vi "OP300ZP_SCANequipements.vi"(8 "Errin":errorcluster caption="errin", 10 "Chaîne":string="Log et conf\\Config.ini", 11 "pathin":path=path "D:/CODE/02 SLIM ZEN") -> (0 "ERROUT":errorcluster caption="error out", 1 "KO?":bool=TRUE, 3 "VISA OUT":T1)   [LabVIEW 2020]
doc: "Ce vi il détecte la presence des équipements"
uses:
  OP300-CONTI-AUTO/VG/VG_ATEQ.vi
  VG/VG_ST5520.vi
  VG/VG_BT3562.vi
  VG/VG_MX5060.vi
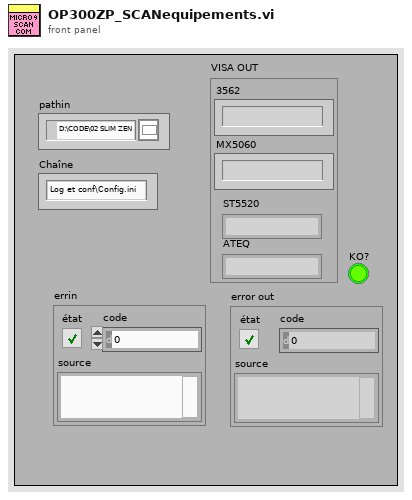
[diagram p1: front panel]
types:
  T1 = cluster{"3562":string, "MX5060":string, "ST5520":string, "ATEQ":string}
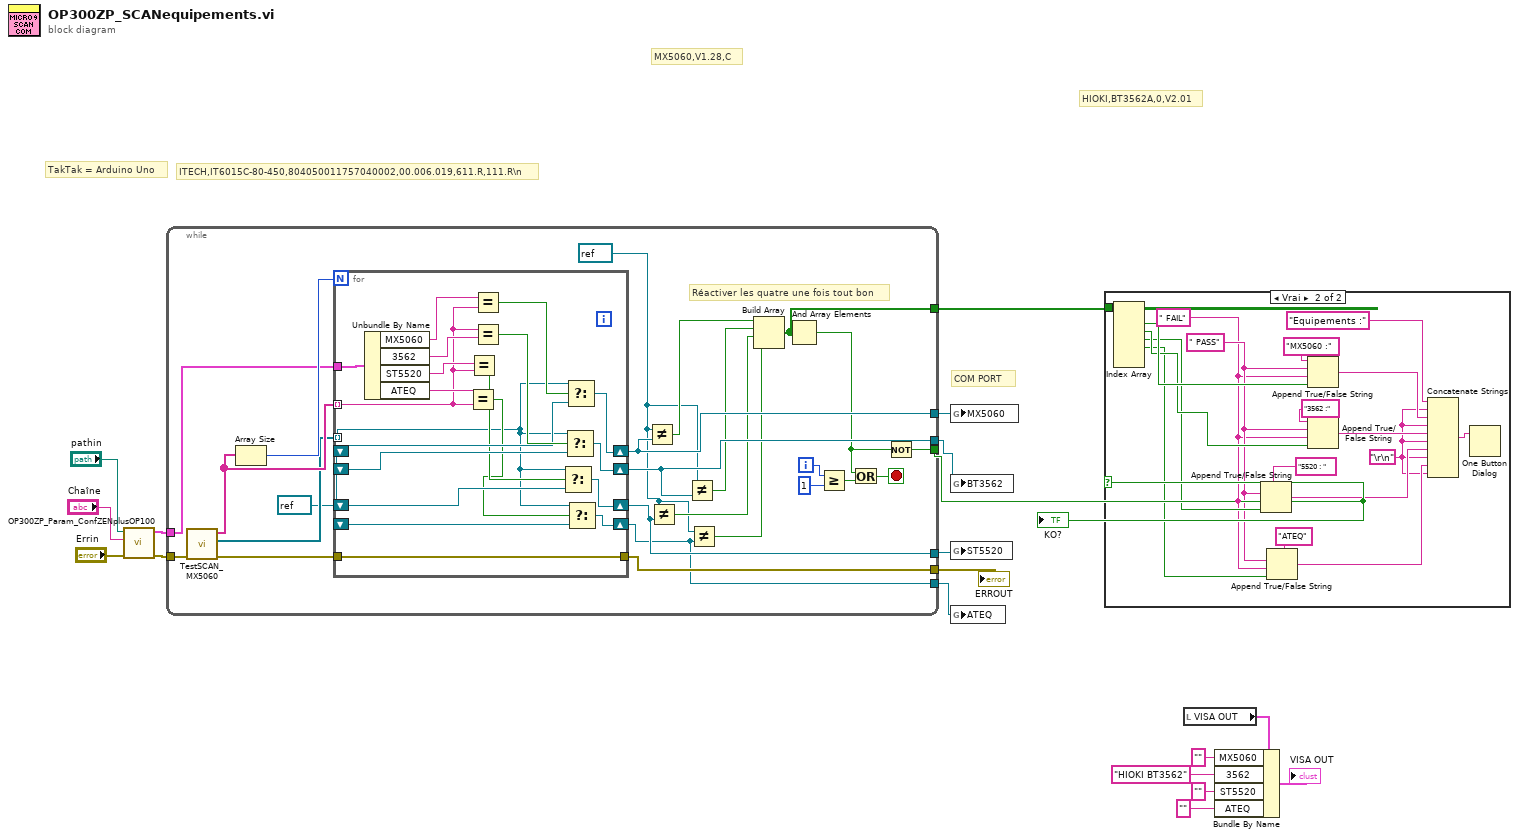
[diagram p0: block diagram]
diagram:
  # "MX5060,V1.28,C"
  # "COM PORT"
  # "HIOKI,BT3562A,0,V2.01"
  # "TakTak = Arduino Uno"
  # "ITECH,IT6015C-80-450,804050011757040002,00.006.019,611.R,111.R\\n"
  n1 = call "OP300ZP_Param_ConfZENplusOP100.vi"("errin"="Errin", "Chaîne"="Chaîne", "pathin"="pathin") -> ("errout"=w15:errorcluster, "VISA OUT"=w14:T1)  [unwired: 7 in]
  n2 = while {
    tunnel: [w32] -> w6
    tunnel: [w31] -> w7
    tunnel: w15 -> [w41]
    tunnel: [w36] -> w18
    tunnel: w14 -> [w33]
    tunnel: [w29] -> w17
    tunnel: [w27] -> w5
    tunnel: [w25] -> w1
    tunnel: [w19] -> w4
    i -> [w35]
    stop <- w38 stop-if-true
    w22 = refnum<visa-resource-name> refnum ("x")
    w28 = refnum<visa-resource-name> refnum ("VISA resource name out")
    # "Réactiver les quatre une fois tout bon"
    n3 = call "TestSCAN_MX5060.vi"("errin"=w41) -> ("error out"=w26:errorcluster, "Tableau 2"=w39:refnum<visa-resource-name>[], "Tableau"=w40:string[])  [unwired: 8 in]
    n4 = Array Size(array=w40) -> (size(s)=w42:i32)
    n5 = for {
      N: w42 -> [_]
      shift-right: [w60] -> w32
      shift-left: w28 -> [w58]
      shift-right: [w59] -> w31
      shift-left: w28 -> [w57]
      tunnel: w40 -> [w47] mode=indexing
      tunnel: w33 -> [w56]
      shift-right: [w53] -> w27
      shift-left: w28 -> [w54]
      tunnel: w39 -> [w45] mode=indexing
      tunnel: w26 -> [w49]
      tunnel: [w49] -> w25
      shift-right: [w44] -> w19
      shift-left: _ -> [w43]
      n6 = Unbundle By Name(w56) -> ("MX5060"=w55:string, "3562"=w50:string, "ST5520"=w52:string, "ATEQ"=w48:string)
      n7 = Equal?(x=w48, y=w47) -> (x = y?=w46:bool)
      n8 = Equal?(x=w52, y=w47) -> (x = y?=w51:bool)
      n9 = Equal?(x=w55, y=w47) -> (x = y?=w61:bool)
      n10 = Equal?(x=w47, y=w50) -> (x = y?=w62:bool)
      n11 = Select(t=w45, s=w51, f=w54) -> (s? t:f=w53:refnum<visa-resource-name>)
      n12 = Select(t=w45, s=w62, f=w57) -> (s? t:f=w59:refnum<visa-resource-name>)
      n13 = Select(t=w45, s=w61, f=w58) -> (s? t:f=w60:refnum<visa-resource-name>)
      n14 = Select(t=w45, s=w46, f=w43) -> (s? t:f=w44:refnum<visa-resource-name>)
    }
    n15 = Not Equal?(x=w22, y=w32) -> (x != y?=w24:bool)
    n16 = Not Equal?(x=w22, y=w27) -> (x != y?=w23:bool)
    n17 = Not Equal?(x=w22, y=w31) -> (x != y?=w21:bool)
    n18 = Not Equal?(x=w22, y=w19) -> (x != y?=w20:bool)
    n19 = Build Array(w24, w21, w23, w20) -> (w29:bool[])
    n20 = And Array Elements(Boolean array=w29) -> (logical AND=w30:bool)
    n21 = Greater Or Equal?(x=w35, y=1) -> (x >= y?=w37:bool)
    n22 = Or(x=w30, y=w37) -> (x .or. y?=w38:bool)
    n23 = Not(x=w30) -> (.not. x?=w36:bool)
  }
  "KO?" <- w18
  "ERROUT" <- w1
  n24 = global write "VG_MX5060.vi" "MX5060"(w6) -> ()
  n25 = global write "VG_BT3562.vi" "BT3562"(w7) -> ()
  n26 = global write "VG_ST5520.vi" "ST5520"(w5) -> ()
  n27 = global write "VG_ATEQ.vi" "ATEQ"(w4) -> ()
  n28 = case shown="Vrai" w18 {
    tunnel: w17 -> [_ w72]
    frame False {
    }
    frame True {
      w63 = "\r\n"
      w67 = " PASS" ("chaîne faux")
      w66 = " FAIL" ("chaîne faux")
      n29 = Index Array(array=w72) -> (element #1=w71:bool, element #2=w70:bool, element #3=w69:bool, element #4=w65:bool)  [unwired: 6 in, 2 out]
      n30 = Append True/False String(1:w69, 2:w66, 3:w67, 4:"5520 : " ("chaîne (\"\")")) -> (0:w74:string)
      n31 = Append True/False String(1:w65, 2:w66, 3:w67, 4:"ATEQ" ("chaîne (\"\")")) -> (0:w64:string)
      n32 = Append True/False String(1:w71, 2:w66, 3:w67, 4:"MX5060 :" ("chaîne (\"\")")) -> (0:w76:string)
      n33 = Append True/False String(1:w70, 2:w66, 3:w67, 4:"3562 :" ("chaîne (\"\")")) -> (0:w75:string)
      n34 = Concatenate Strings("Equipements :" ("chaîne"), w63, w76, w63, w75, w63, w74, w63, w64, w63) -> (w73:string)
      n35 = One Button Dialog(message=w73) -> ()  [unwired: 1 in, 1 out]
    }
  }
  n36 = local read "VISA OUT"() -> (w10:T1)
  n37 = Bundle By Name(cluster=w10, "MX5060"="", "3562"="HIOKI BT3562", "ST5520"="", "ATEQ"="") -> (→"VISA OUT":T1)
